vi "Configure Output Range and Manual Value.vi"(0 "VISA resource name":refnum<visa-resource-name>, 5 "Heater Output (1:1)":u16(ring)=1 items=["1"=1, "2"=2], 7 "Range (0:Off)":u16(ring) items=["Off", "Low (On)", "Medium", "High"], 9 "Manual Output (0.00 %)":dbl format="%.2f", 11 "error in (no error)":errorcluster) -> (4 "VISA resource name out":refnum<visa-resource-name>, 15 "error out":errorcluster)   [LabVIEW 2015, in "Lake Shore 335.lvlib"]
doc: "Configures the Range and Manual Output settings for both heater outputs."
uses:
  <instrlib>/Lake Shore 335/Lake Shore 335.lvlib
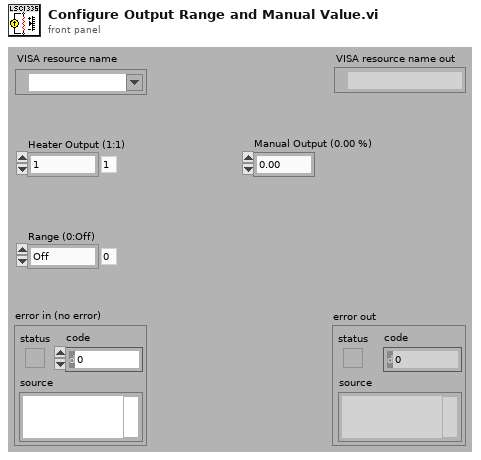
[diagram p1: front panel]
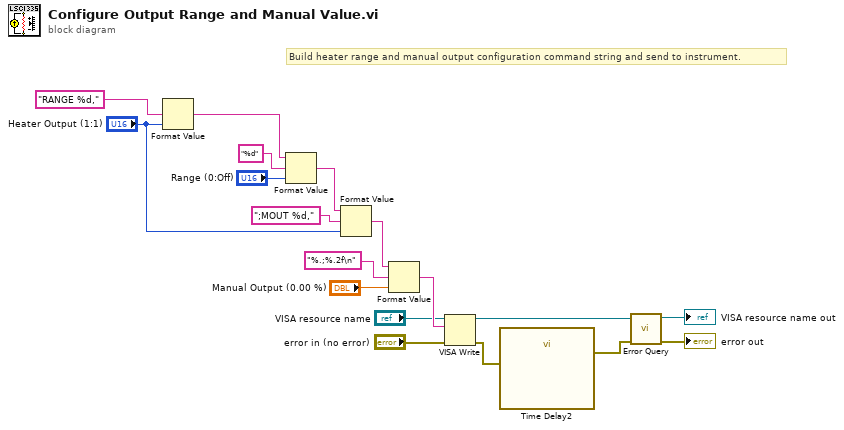
[diagram p0: block diagram]
diagram:
  # "Build heater range and manual output configuration command string and send to instrument."
  n1 = Format Value(format string="RANGE %d,", value (0)="Heater Output (1:1)") -> (output string=w14:string)  [unwired: 1 in]
  n2 = Format Value(string ("")=w14, format string="%d", value (0)="Range (0:Off)") -> (output string=w13:string)
  n3 = Format Value(string ("")=w13, format string=";MOUT %d,", value (0)="Heater Output (1:1)") -> (output string=w1:string)
  n4 = Format Value(string ("")=w1, format string="%.;%.2f\n", value (0)="Manual Output (0.00 %)") -> (output string=w8:string)
  n5 = VISA Write(VISA resource name="VISA resource name", write buffer=w8, error in (no error)="error in (no error)") -> (VISA resource name out=w9:refnum<visa-resource-name>, error out=w11:errorcluster)  [unwired: 1 out]
  n6 = call "Time Delay2"("error in (no error)"=w11) -> ("error out"=w10:errorcluster)  [unwired: 10 in]
  n7 = call <instrlib>:"Error Query.vi"("error in (no error)"=w10, "VISA resource name"=w9) -> ("error out"=→"error out":errorcluster, "VISA resource name out"=→"VISA resource name out":refnum<visa-resource-name>)  [unwired: 7 in, 1 out]
